vi "globalSetUp.vi"(8 "error in":errorcluster, 11 "Single Board Loopback in":refnum<class "Single Board Loopback.lvclass">) -> (0 "error out":errorcluster, 3 "Single Board Loopback out":refnum<class "Single Board Loopback.lvclass">)   [LabVIEW 2024, in "Single Board Loopback.lvclass"]
uses:
  Single Board Loopback.lvclass
  Single Board Loopback.lvclass/Single Board Loopback.ctl
  <vilib>/NI/VeriStand Custom Device Testing Tools/VeriStandTestUtilities/VeriStandTestUtilities.lvlib
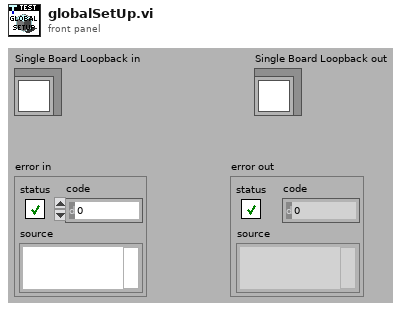
[diagram p1: front panel]
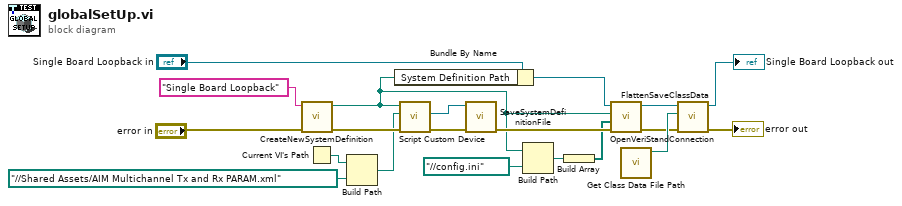
[diagram p0: block diagram]
diagram:
  n1 = call <vilib>:"CreateNewSystemDefinition.vi"("error in"="error in", "System Definition Name"="Single Board Loopback" ("Channel")) -> ("error out"=w16:errorcluster, "System Definition Path"=w2:path)  [unwired: 8 in]
  n2 = Current VI's Path() -> (path=w20:path)
  n3 = Build Path(base path=w20, name or relative path=path "../../Shared Assets/AIM Multichannel Tx and Rx PARAM.xml") -> (appended path=w13:path)
  n4 = Bundle By Name(cluster="Single Board Loopback in", "System Definition Path"=w2) -> (w4:refnum<class "Single Board Loopback.lvclass">)
  n5 = call "Script Custom Device.vi"("error in"=w16, "Parameter File Path"=w13, "System Definition File Path In"=w2) -> ("error out"=w19:errorcluster, "System Definition Reference"=w14:refnum<k24>)  [unwired: 5 in, 2 out]
  n6 = call <vilib>:"SaveSystemDefinitionFile.vi"("error in (no error)"=w19, "System Definition Reference in"=w14) -> ("error out"=w15:errorcluster)  [unwired: 8 in, 1 out]
  n7 = Build Path(base path=w2, name or relative path=path "../../config.ini" ("overrides files")) -> (appended path=w8:path)
  n8 = Build Array(w8) -> (w7:path[])
  n9 = call-dynamic "OpenVeriStandConnection.vi"("error in (no error)"=w15, "overrides files"=w7, "System Definition File"=w2, "VeriStand Test Case in"=w4) -> ("error out"=w5:errorcluster, "VeriStand Test Case out"=w1:refnum<class "Single Board Loopback.lvclass">)  [unwired: 5 in, 1 out]
  n10 = call "Get Class Data File Path.vi"() -> ("Class Data File Path"=w6:path)  [unwired: 11 in]
  n11 = call-dynamic "FlattenSaveClassData.vi"("error in"=w5, "Class Data File Path"=w6, "VeriStandTestCase in"=w1) -> ("error out"=→"error out":errorcluster, "VeriStandTestCase out"=→"Single Board Loopback out":refnum<class "Single Board Loopback.lvclass">)  [unwired: 7 in]
